vi "SetParamValue.vi"(4 "ID":u16, 6 "plValue":i32, 7 "ZWO num":i32, 9 "Cluster":T1, 10 "Boolean":bool, 11 "ZWO_ASI in":refnum<class "ZWO_ASI.lvclass">) -> (3 "Parameter List":T2(array[cluster]))   [LabVIEW 2023, in "ZWO_ASI.lvlib" / "ZWO_ASI.lvclass"]
uses:
  ZWO_ASI.lvclass
  Labview_ASI_demo_64bit_221128/user.lib/ASICamera2_no_err/ASICamera2_no_err.lvlib
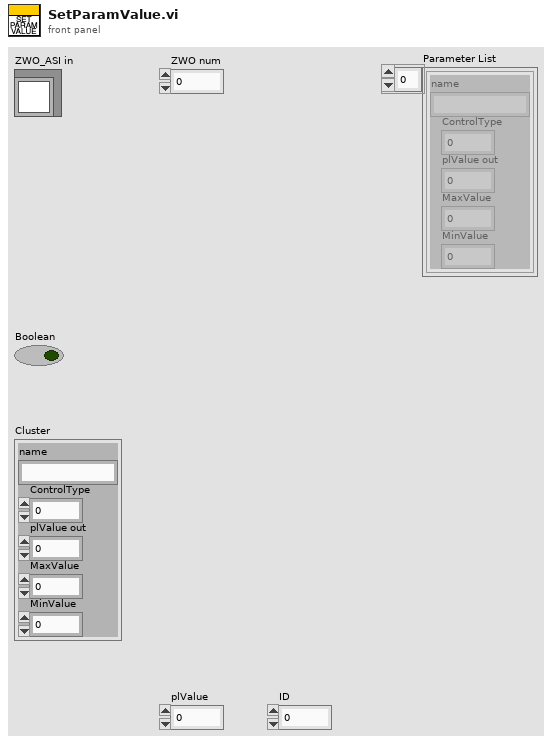
[diagram p1: front panel]
types:
  T1 = cluster{"name":string, "ControlType":u32, "plValue out":i32, "MaxValue":i32, "MinValue":i32}
  T2 = cluster{"name":string, "ControlType":u32, "plValue out":i32, "MaxValue":i32, "MinValue":i32}[]
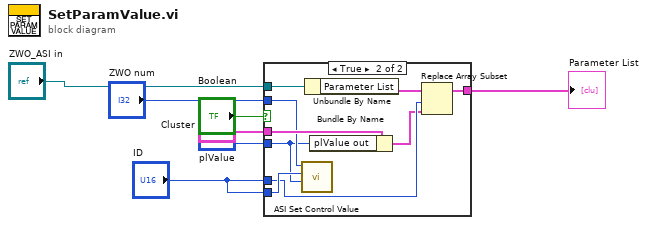
[diagram p0: block diagram]
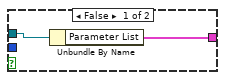
[diagram p2: hidden frame]
diagram:
  n1 = case shown="True" "Boolean" {
    tunnel: "ID" -> [_ w17]
    tunnel: "plValue" -> [_ w15]
    tunnel: "Cluster" -> [_ w18]
    tunnel: "ZWO num" -> [_ w16]
    tunnel: "ID" -> [_ w14]
    tunnel: [w9 w12] -> w6
    tunnel: "ZWO_ASI in" -> [w8 w11]
    frame False {
      n2 = Unbundle By Name(w8) -> ("Parameter List"=w9:T2)
    }
    frame True {
      n3 = call "ASI Set Control Value.vi"("lValue"=w15, "ControlType"=w17, "iCameraID"=w16) -> ()  [unwired: 8 in, 1 out]
      n4 = Unbundle By Name(w11) -> ("Parameter List"=w10:T2)
      n5 = Bundle By Name(cluster=w18, "plValue out"=w15) -> (w13:T1)
      n6 = Replace Array Subset(array=w10, new element=w13, index=w14) -> (w12:T2)
    }
  }
  "Parameter List" <- w6
